vi "ChkSync.vi"(9 "ConfigReg":refnum<vi>, 11 "Msg":string) -> ()   [LabVIEW 2025]
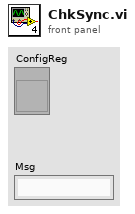
[diagram p1: front panel]
types:
  T1 = typedef "Config.ctl" = cluster{"Pico":refnum<visa-resource-name>, "Range":T2, "Mode":T3, "R":dbl[]}
  T2 = typedef "Range.ctl" = enum16{"0.26", "0.52", "1.03", "2.05", "4.1", "6.2"}
  T3 = typedef "Mode.ctl" = enum16{"R1 Only", "Parallel", "Serial"}
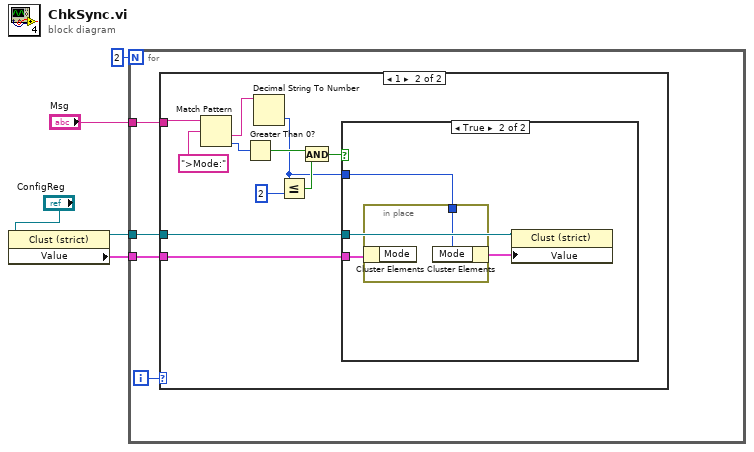
[diagram p0: block diagram]
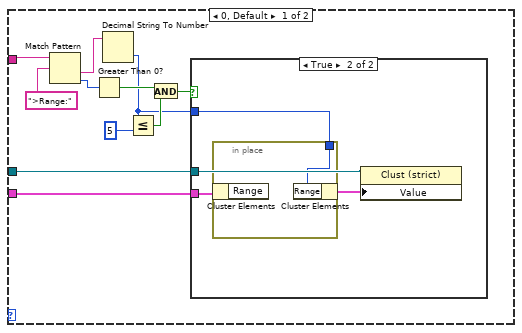
[diagram p2: hidden frame]
diagram:
  n1 = property class="Clust (strict)"(reference="ConfigReg") -> (reference out=w1:refnum<vi>, "Value"=w2:T1)  [unwired: 1 in, 1 out]
  n2 = for {
    N: 2 -> [_]
    tunnel: "Msg" -> [w8]
    tunnel: w2 -> [w7]
    tunnel: w1 -> [w6]
    i -> [w9]
    n3 = case shown="1" w9 {
      tunnel: w8 -> [w20 w36]
      tunnel: w7 -> [w17 w33]
      tunnel: w6 -> [w16 w32]
      frame 0, Default {
        n4 = Match Pattern(string=w20, regular expression=">Range:" ("y")) -> (after substring=w10:string, offset past match=w18:i32)  [unwired: 1 in, 2 out]
        n5 = Greater Than 0?(x=w18) -> (x > 0?=w13:bool)
        n6 = Decimal String To Number(string=w10) -> (number=w11:i32)  [unwired: 2 in, 1 out]
        n7 = Less Or Equal?(x=w11, y=5) -> (x <= y?=w12:bool)
        n8 = And(x=w13, y=w12) -> (x .and. y?=w14:bool)
        n9 = case shown="True" w14 {
          tunnel: w17 -> [_ w24]
          tunnel: w16 -> [_ w23]
          tunnel: w11 -> [_ w21]
          frame False {
          }
          frame True {
            n10 = in-place {
              in-place-border: w21 -> [w25]
              n11 = in-place-cluster #1(w24) -> ()  [unwired: 1 out]
              n12 = in-place-cluster #1("Range"=w25) -> (w22:T1)
            }
            n13 = property class="Clust (strict)"(reference=w23, "Value"=w22) -> ()  [unwired: 1 in, 2 out]
          }
        }
      }
      frame 1 {
        n14 = Match Pattern(string=w36, regular expression=">Mode:" ("y")) -> (after substring=w26:string, offset past match=w34:i32)  [unwired: 1 in, 2 out]
        n15 = Greater Than 0?(x=w34) -> (x > 0?=w29:bool)
        n16 = Decimal String To Number(string=w26) -> (number=w27:i32)  [unwired: 2 in, 1 out]
        n17 = Less Or Equal?(x=w27, y=2) -> (x <= y?=w28:bool)
        n18 = And(x=w29, y=w28) -> (x .and. y?=w30:bool)
        n19 = case shown="True" w30 {
          tunnel: w33 -> [_ w40]
          tunnel: w32 -> [_ w39]
          tunnel: w27 -> [_ w37]
          frame False {
          }
          frame True {
            n20 = in-place {
              in-place-border: w37 -> [w41]
              n21 = in-place-cluster #2(w40) -> ()  [unwired: 1 out]
              n22 = in-place-cluster #2("Mode"=w41) -> (w38:T1)
            }
            n23 = property class="Clust (strict)"(reference=w39, "Value"=w38) -> ()  [unwired: 1 in, 2 out]
          }
        }
      }
    }
  }
